vi "Claim Core.vi"(8 "error in":errorcluster, 10 "Device ID":string, 11 "Spark Reference In":T1) -> (0 "error out":errorcluster, 2 "Function Response":T4, 3 "Spark Reference Out":T1)   [LabVIEW 2014, in "Spark API.lvlib"]
doc: "Request that a given Spark device be registered to the currently connected Spark IO account."
uses:
  Spark API.lvlib
  Controls/Spark Reference.ctl
  <vilib>/httpClient/ClientHandle.ctl
  Controls/Device Query JSON.ctl
  Controls/Function Response JSON.ctl
  <vilib>/httpClient/POSTBuffer.vi
  <vilib>/httpClient/LabVIEWHTTPClient.lvlib
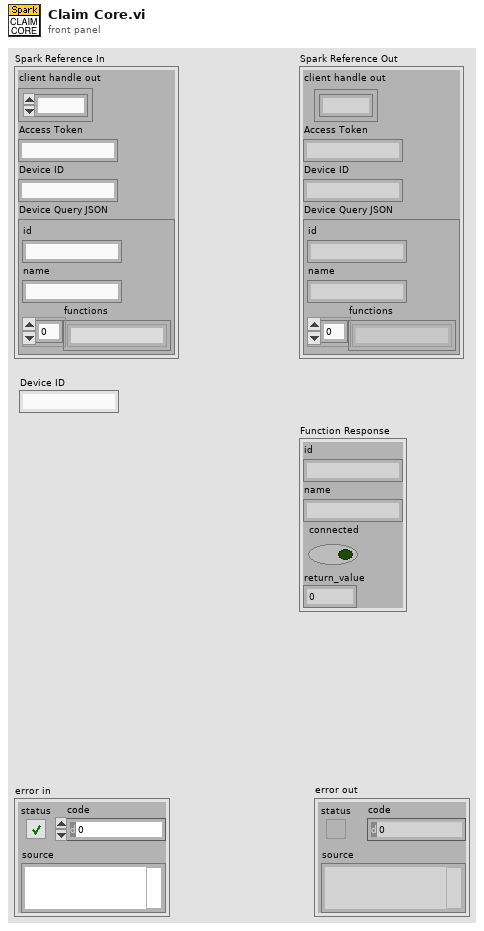
[diagram p1: front panel]
types:
  T1 = typedef "Spark API.lvlib/Spark Reference.ctl" = cluster{"client handle out":T2, "Access Token":string, "Device ID":string, "Device Query JSON":T3}
  T2 = typedef "LabVIEWHTTPClient.lvlib/ClientHandle.ctl" = refnum<k1>
  T3 = typedef "Spark API.lvlib/Device Query JSON.ctl" = cluster{"id":string, "name":string, "functions":string[]}
  T4 = typedef "Spark API.lvlib/Function Response JSON.ctl" = cluster{"id":string, "name":string, "connected":bool, "return_value":dbl}
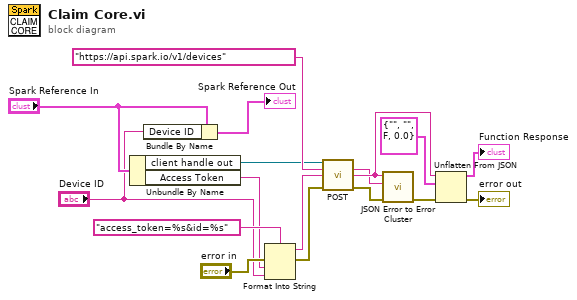
[diagram p0: block diagram]
diagram:
  n1 = Unbundle By Name("Spark Reference In") -> ("client handle out"=w13:T2, "Access Token"=w1:string)
  n2 = Bundle By Name(cluster="Spark Reference In", "Device ID"="Device ID") -> (→"Spark Reference Out":T1)
  n3 = Format Into String(format string="access_token=%s&id=%s", error in="error in", w1, "Device ID") -> (resulting string=w11:string, error out=w8:errorcluster)  [unwired: 1 in]
  n4 = call-poly <vilib>:"POST.vi"("client handle"=w13, "url"="https://api.spark.io/v1/devices", "buffer"=w11, "error in (no error)"=w8) -> ("headers"=w5:string, "body"=w6:string, "error out"=w10:errorcluster)  [unwired: 8 in, 1 out]
  n5 = call "JSON Error to Error Cluster.vi"("error in (no error)"=w10, "headers"=w5, "JSON string"=w6) -> ("error out"=w7:errorcluster)  [unwired: 8 in]
  n6 = Unflatten From JSON(JSON string=w6, type and defaults=T4 {"id"="", "name"="", "connected"=FALSE, "return_value"=0.0} ("Function Response"), error in (no error)=w7) -> (value=→"Function Response":T4, error out=→"error out":errorcluster)  [unwired: 4 in]
